vi "LV GET REGISTER.vi"(9 "Board Handle In":T1, 11 "Name":string) -> (0 "Result code":i32, 1 "Board Handle Out":T1, 3 "Value":u32)   [LabVIEW 2021]
uses:
  SciSDK_Labview.lvlib
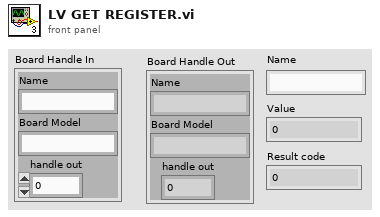
[diagram p1: front panel]
types:
  T1 = cluster{"Name":string, "Board Model":string, "handle out":u64}
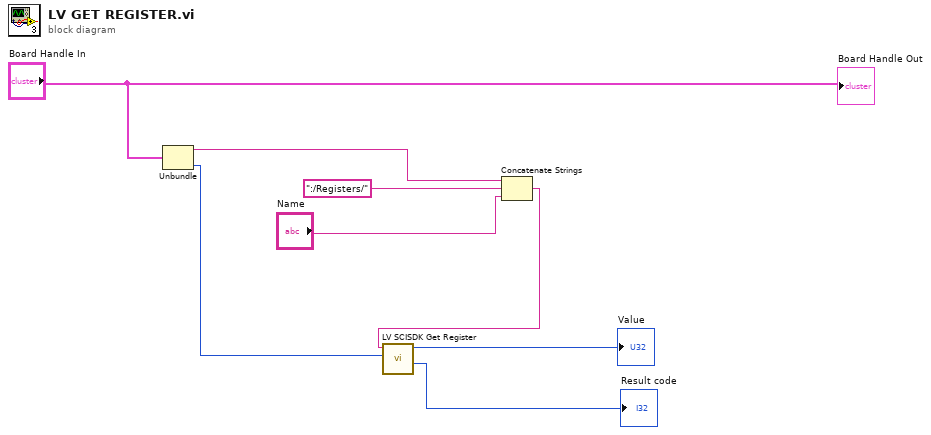
[diagram p0: block diagram]
diagram:
  n1 = Unbundle("Board Handle In") -> ("Name"=w7:string, "handle out"=w2:u64)  [unwired: 1 out]
  n2 = Concatenate Strings(w7, ":/Registers/" ("string"), "Name") -> (w4:string)
  n3 = call "LV SCISDK Get Register.vi"("handle"=w2, "Path"=w4) -> ("function return"=→"Result code":i32, "value"=→"Value":u32)  [unwired: 6 in, 2 out]
  "Board Handle Out" <- "Board Handle In"
